vi "controller_simulator.vi"() -> ()   [LabVIEW 2010]
uses:
  space_vector_cluster.ctl
panel:
  in  "command mode":enum16{"step", "absolute"}(ring)
  in  "perform motion?":bool
  in  "motion trigger":bool
  in  "current position":T1
  in  "command":T1
  out "loop counter":i32
  in  "stop":bool
  # "Simulator of an external stage controller"
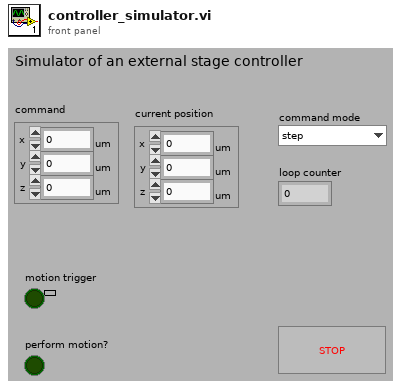
[diagram p1: front panel]
types:
  T1 = typedef "space_vector_cluster.ctl" = cluster{"x":dbl[unit], "y":dbl[unit], "z":dbl[unit]}
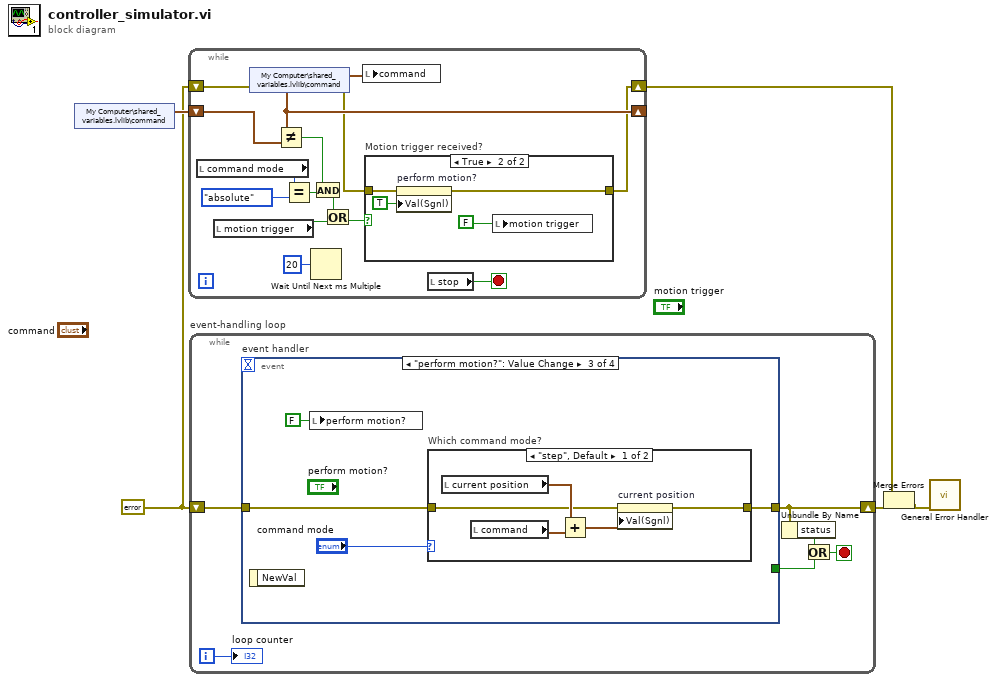
[diagram p0: block diagram]
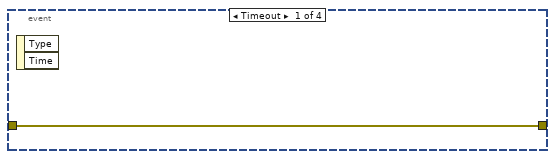
[diagram p3: hidden frame]
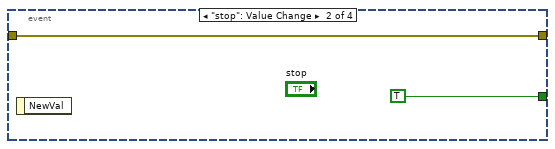
[diagram p4: hidden frame]
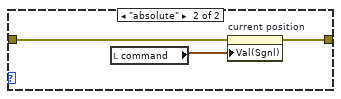
[diagram p5: hidden frame]
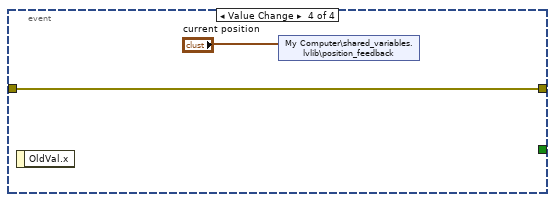
[diagram p6: hidden frame]
diagram:
  w1 = errorcluster {"status"=FALSE, "code"=0, "source"=""} ("error IO")
  n1 = shared-variable "My Computer\\shared_variables.lvlib\\command"() -> (w5:T1)  [unwired: 1 in, 1 out]
  n2 = while {
    shift-right: [w15] -> _
    shift-left: w5 -> [w17]
    shift-right: [w12] -> w2
    shift-left: w1 -> [w14]
    stop <- w19 stop-if-true
    n3 = local read "command mode"() -> (w11:enum16{"step", "absolute"})
    n4 = local read "motion trigger"() -> (w6:bool)
    n5 = shared-variable "My Computer\\shared_variables.lvlib\\command"(error in=w14) -> (w15:T1, error out=w13:errorcluster)
    n6 = Not Equal?(x=w15, y=w17) -> (x != y?=w8:bool)
    n7 = Equal?(x=w11, y=enum16{"step", "absolute"}."absolute") -> (x = y?=w9:bool)
    n8 = Wait Until Next ms Multiple(millisecond multiple=u32 20) -> ()  [unwired: 1 out]
    n9 = And(x=w8, y=w9) -> (x .and. y?=w7:bool)
    n10 = Or(x=w7, y=w6) -> (x .or. y?=w16:bool)
    n11 = local write "command"(w15) -> ()
    n12 = case "Motion trigger received?" shown="True" w16 {
      tunnel: w13 -> [w20 w23]
      tunnel: [w20 w22] -> w12
      frame False {
      }
      frame True {
        n13 = property on="perform motion?" class="Bool (strict)"(error in=w23, "Val(Sgnl)"=TRUE ("Value (Signaling)")) -> (error out=w22:errorcluster)  [unwired: 1 in, 1 out]
        n14 = local write "motion trigger"(FALSE) -> ()
      }
    }
    n15 = local read "stop"() -> (w19:bool)
  }
  n16 = while "event-handling loop" {
    shift-right: [w27] -> w4
    shift-left: w1 -> [w25]
    i -> [w26]
    stop <- w29 stop-if-true
    n17 = event "event handler" shown="[2] \"perform motion?\": Value Change" {
      selector: _ -> [_ _ _ _]
      dyn-events: _ -> [_ _ _ _]
      timeout: _ -> [_ _ _ _]
      tunnel: [_ TRUE _ _] -> w28
      tunnel: [w31 w32 w34 w46] -> w27
      tunnel: w25 -> [w31 w32 w35 w46]
      event Timeout {
        n18 = event-data() -> ()  [unwired: 1 in, 2 out]
      }
      event "stop": Value Change {
        n19 = event-data() -> ()  [unwired: 1 in, 1 out]
      }
      event "perform motion?": Value Change {
        n20 = event-data() -> ()  [unwired: 1 in, 1 out]
        n21 = local write "perform motion?"(FALSE ("perform motion?")) -> ()
        n22 = case "Which command mode?" shown="\"step\", Default" "command mode" {
          tunnel: w35 -> [w39 w45]
          tunnel: [w38 w44] -> w34
          frame "step", Default {
            n23 = local read "current position"() -> (w41:T1)
            n24 = local read "command"() -> (w42:T1)
            n25 = Add(x=w41, y=w42) -> (x+y=w40:T1)
            n26 = property on="current position" class="Clust (strict)"(error in=w39, "Val(Sgnl)"=w40) -> (error out=w38:errorcluster)  [unwired: 1 in, 1 out]
          }
          frame "absolute" {
            n27 = local read "command"() -> (w43:T1)
            n28 = property on="current position" class="Clust (strict)"(error in=w45, "Val(Sgnl)"=w43) -> (error out=w44:errorcluster)  [unwired: 1 in, 1 out]
          }
        }
      }
      event Value Change {
        n29 = event-data() -> ()  [unwired: 1 in, 1 out]
        n30 = shared-variable "My Computer\\shared_variables.lvlib\\position_feedback"("current position") -> ()  [unwired: 1 in, 1 out]
      }
    }
    n31 = Unbundle By Name(w27) -> ("status"=w30:bool)
    n32 = Or(x=w30, y=w28) -> (x .or. y?=w29:bool)
    "loop counter" <- w26
  }
  n33 = Merge Errors(w2, w4) -> (w3:errorcluster)
  n34 = call <vilib>:"General Error Handler.vi"("error in (no error)"=w3) -> ()  [unwired: 10 in, 5 out]
